vi "main_v1.1.vi"() -> ()   [LabVIEW 2012]
uses:
  SensorSettingCtl.ctl
  SensorTypes.ctl
  states.ctl
  globalVariables.vi
  <vilib>/Analysis/baseanly.llb/Mean (DBL).vi
  <vilib>/Analysis/NI_AALBase.lvlib
panel:
  in  "endindices":i32[](array[numeric])
  in  "startindices":i32[](array[numeric])
  in  "cancel button data analysis":bool
  out "XY Graph 11":cluster{dbl[], dbl[]}[](graph)
  out "XY Graph 10":cluster{dbl[], dbl[]}[](graph)
  out "size":i32[](array[numeric])
  out "sum":dbl[](array[numeric])
  out "XY Graph 9":cluster{dbl[], dbl[]}[](graph)
  out "XY Graph 8":cluster{dbl[], dbl[]}[](graph)
  out "meas. time / s":dbl format="%#.1f"
  out "diff chg":dbl
  out "charges":dbl[](array[numeric])
  out "times":dbl[](array[numeric])
  out "diff":dbl
  in  "max. meas. time / s":dbl=3000.0
  out "mean currents":dbl[](array[numeric])
  out "measuring":bool
  out "i_e":i32
  out "i_s":i32
  out "XY Graph raw":cluster{dbl[], dbl[]}[](graph)
  out "XY Graph":cluster{dbl[], dbl[]}[](graph)
  in  "size of buffer":i32=1000000
  in  "Path for measuring results":path=path "C:/Users/Induelec/Desktop/test_output"
  in  "Sensor types":T1[](array[typedef])=[enum."ITL 900 (Analogue)", enum."CAB 300-C SP3 (CAN)", enum."xyz TODO (PWM)", enum."xyz TODO (LIN)", enum."xyz TODO (Analogue)"]
  in  "Sensor-enabling":T2[](array[typedef])=[{"VISA resource name"="", "use sensor"=FALSE}, {"VISA resource name"="", "use sensor"=TRUE}, {"VISA resource name"="", "use sensor"=FALSE}, {"VISA resource name"="", "use sensor"=FALSE}, {"VISA resource name"="", "use sensor"=FALSE}]
  in  "cancel button":bool
  in  "start Button":bool
  out "Error Flag":bool
  # "Measurement of Current Sensors from LEM"
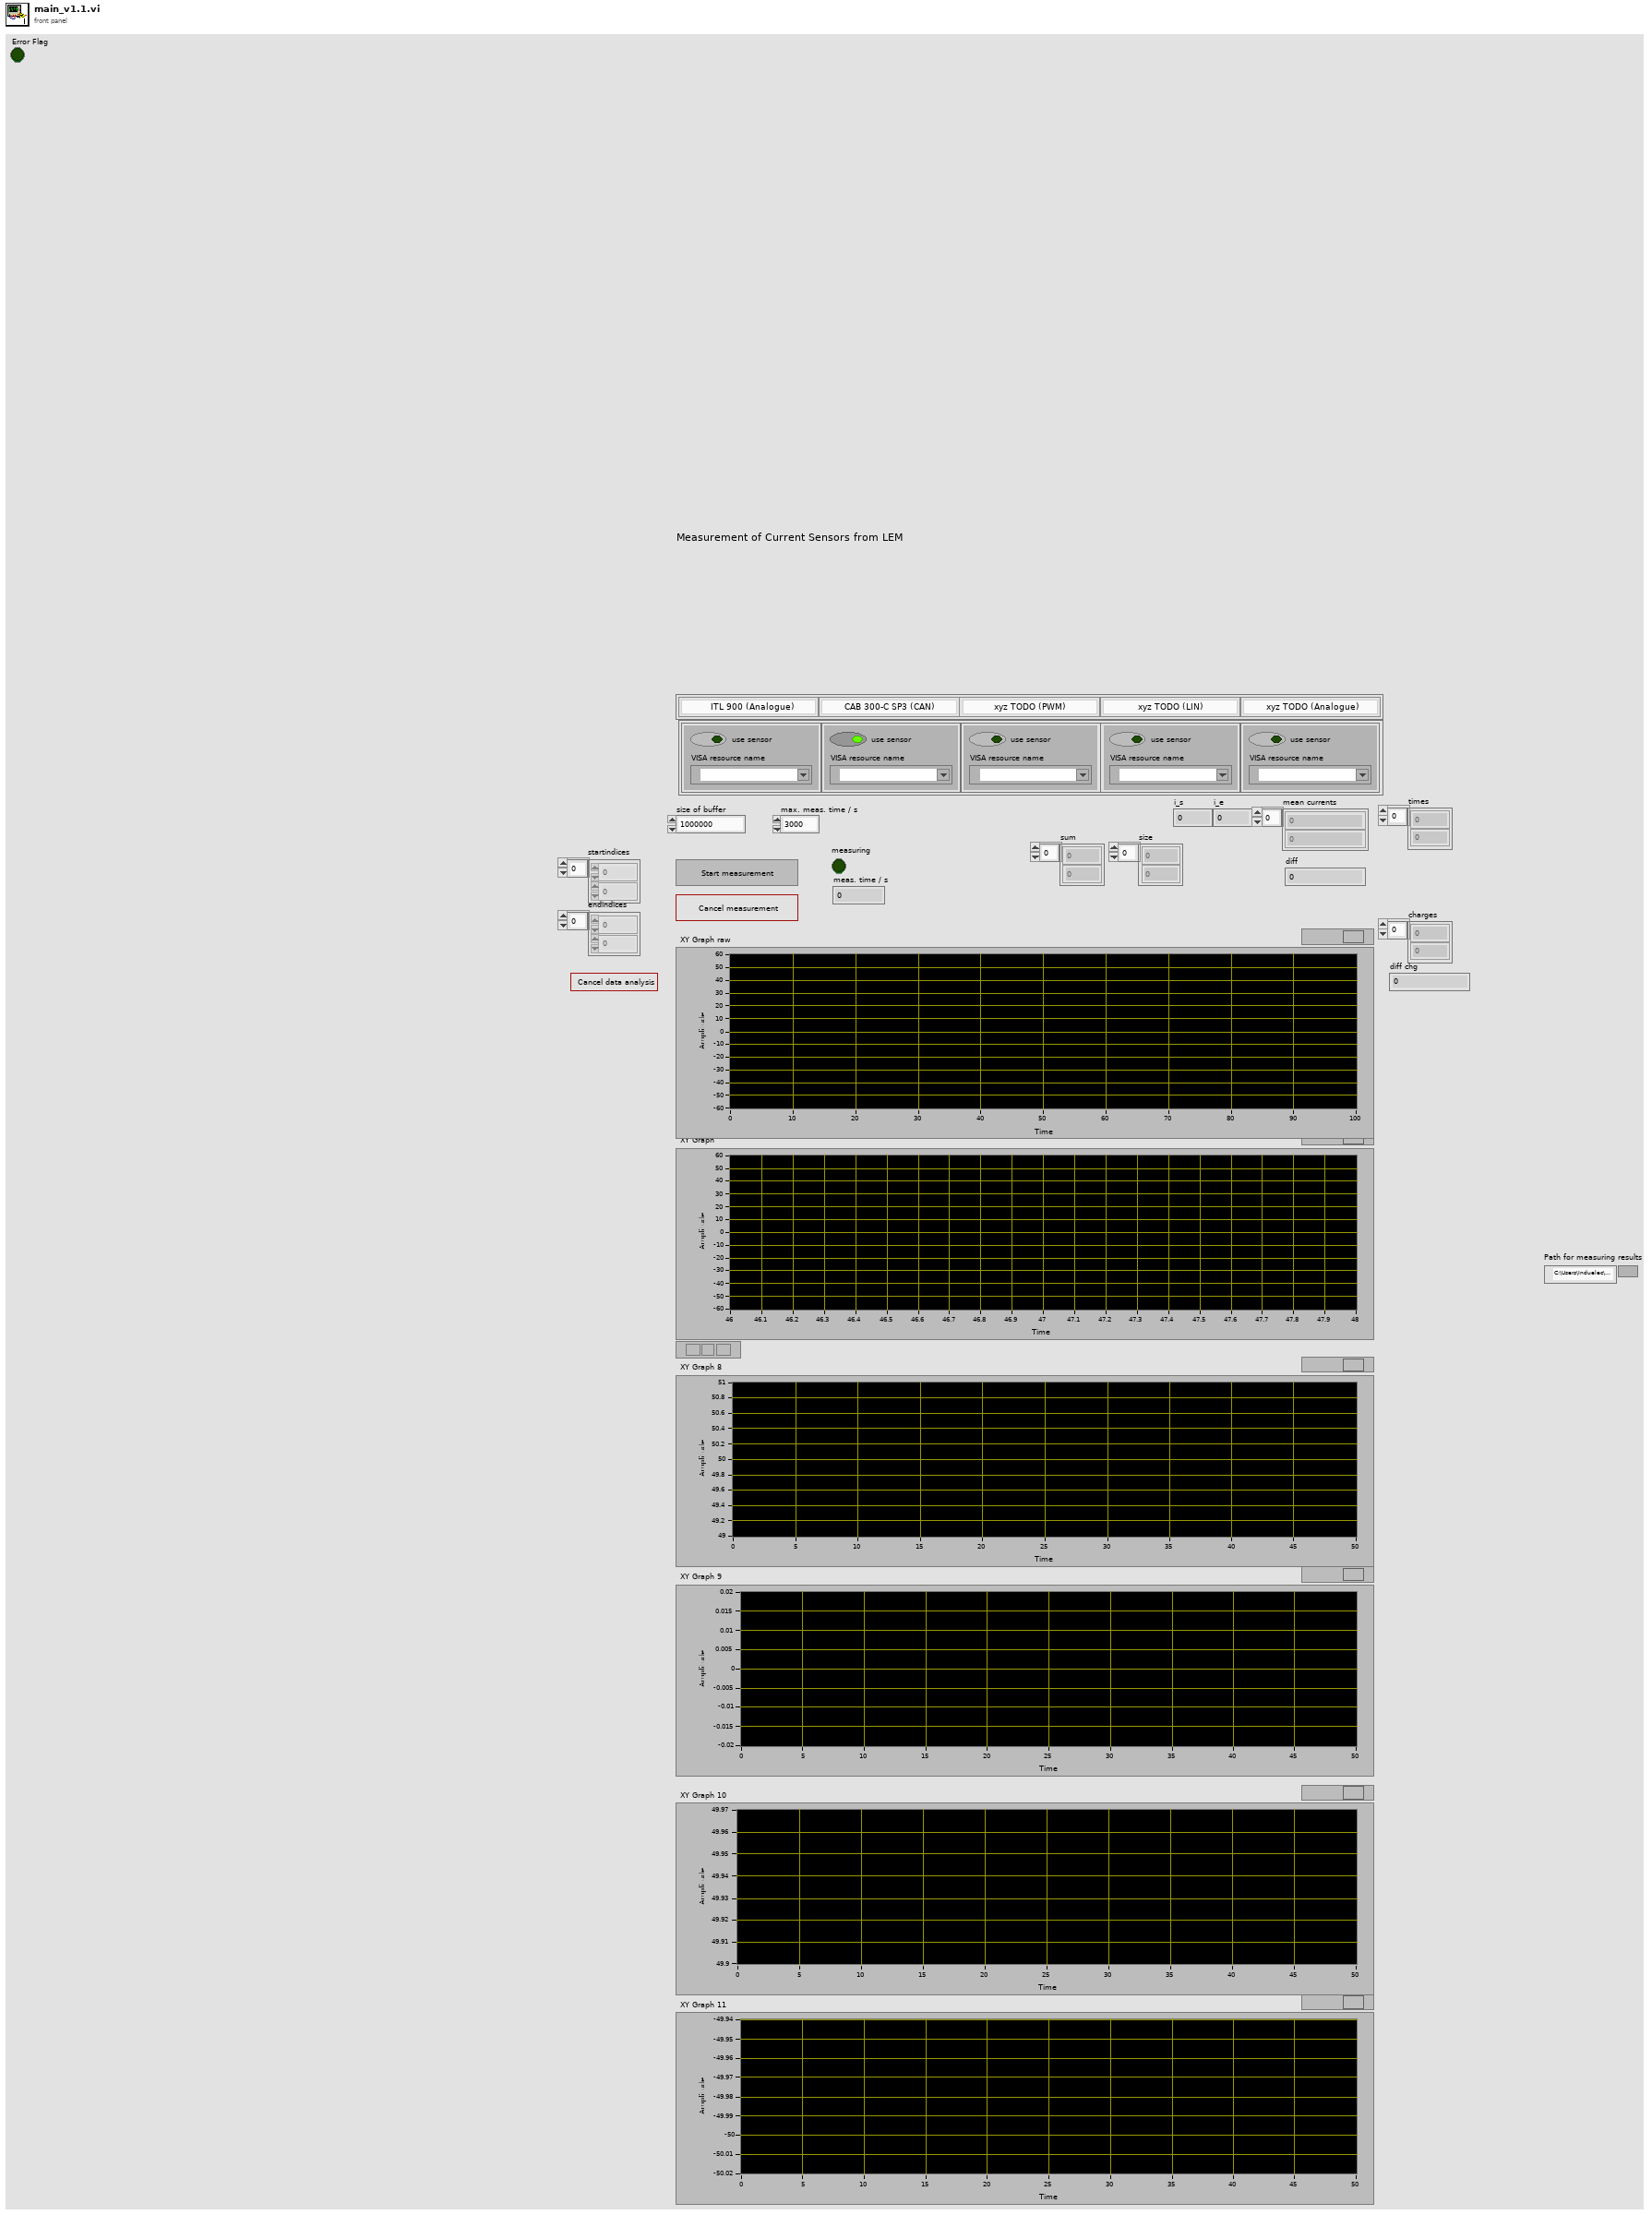
[diagram p1: front panel]
types:
  T1 = typedef "SensorTypes.ctl" = enum16{"ITL 900 (Analogue)", "CAB 300-C SP3 (CAN)", "xyz TODO (PWM)", "xyz TODO (LIN)", "xyz TODO (Analogue)"}
  T2 = typedef "SensorSettingCtl.ctl" = cluster{"VISA resource name":refnum<visa-resource-name>, "use sensor":bool}
  T3 = typedef "states.ctl" = enum16{"init", "wait for user confirm", "start sensors", "measure", "data analysis", "terminate"}
  T4 = typedef "Semaphore RefNum" = refnum<k1>
  T5 = typedef "TimeValue.ctl" = cluster{"Time of measurement":timestamp, "Current value":dbl}
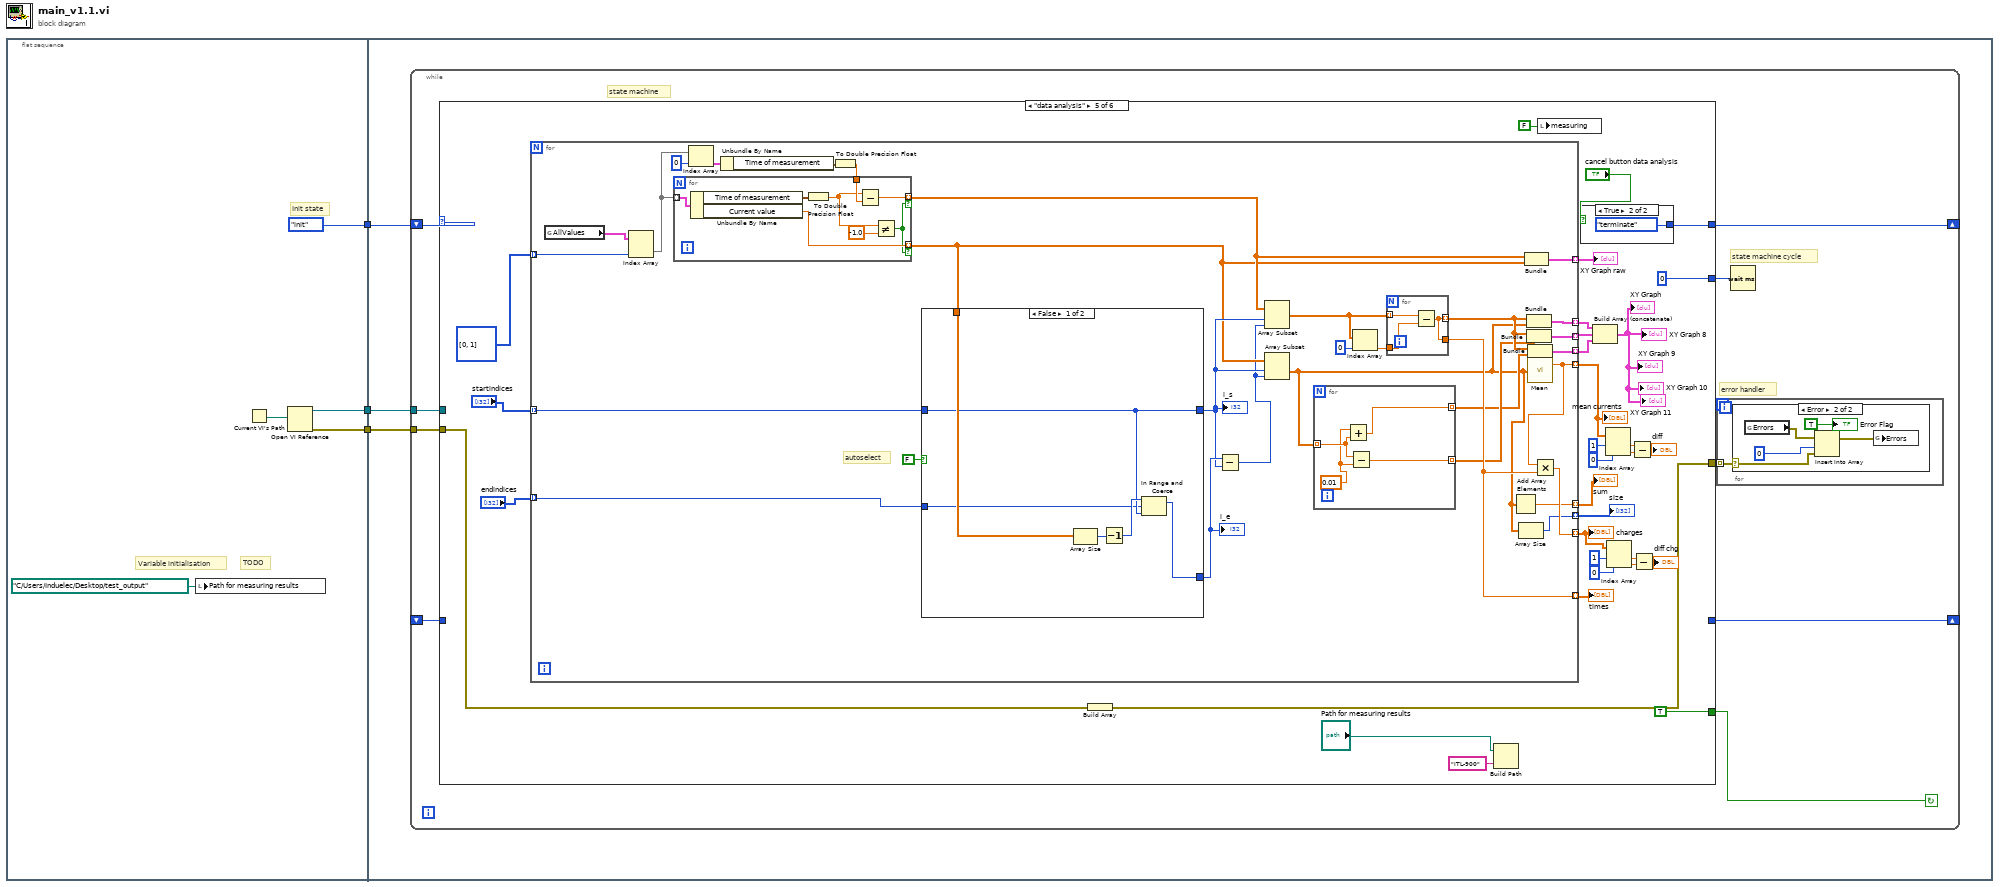
[diagram p0: block diagram]
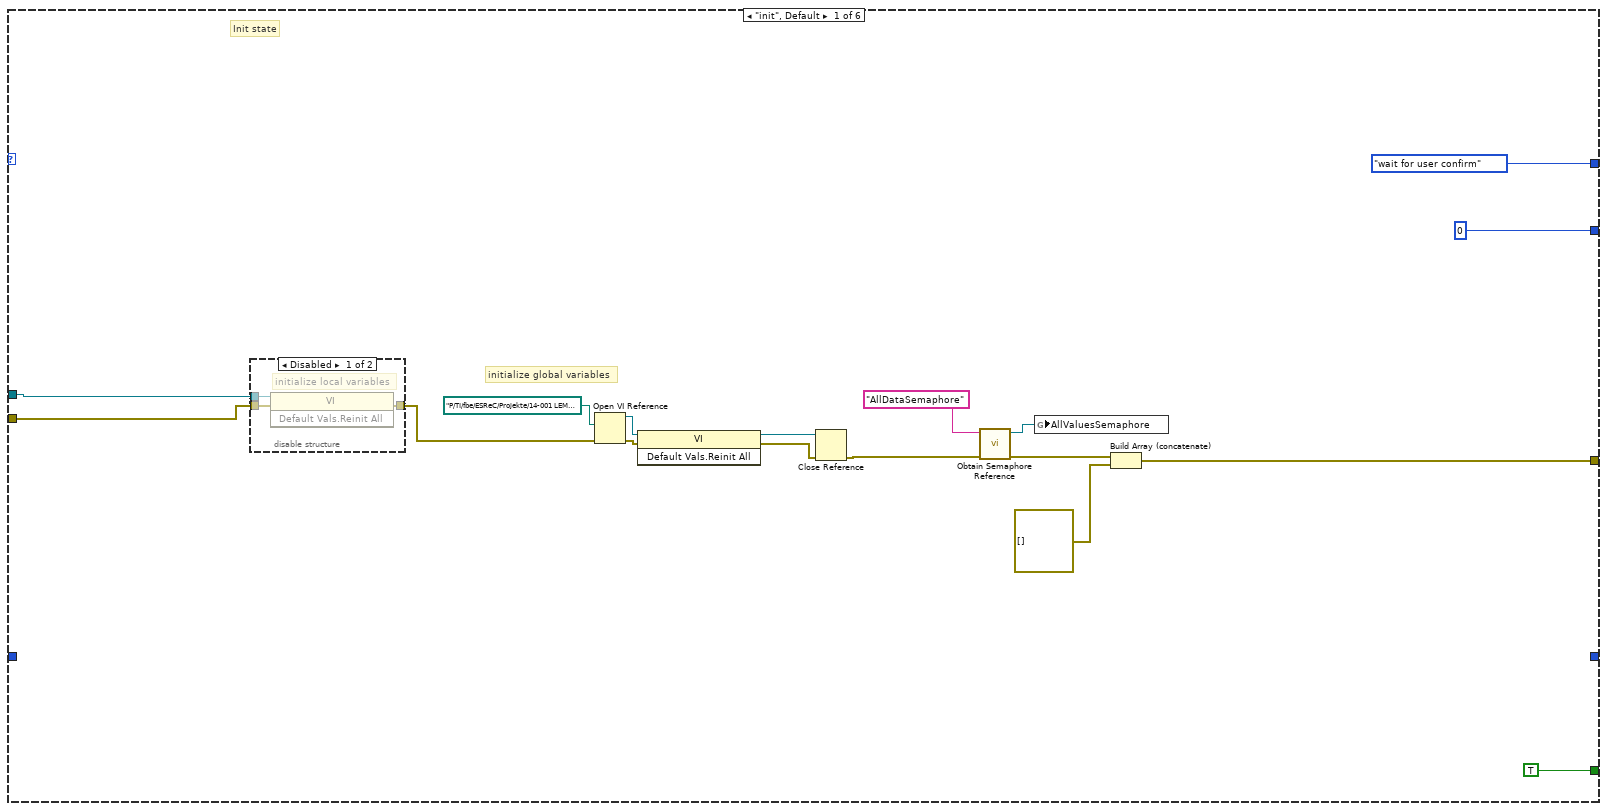
[diagram p3: hidden frame]
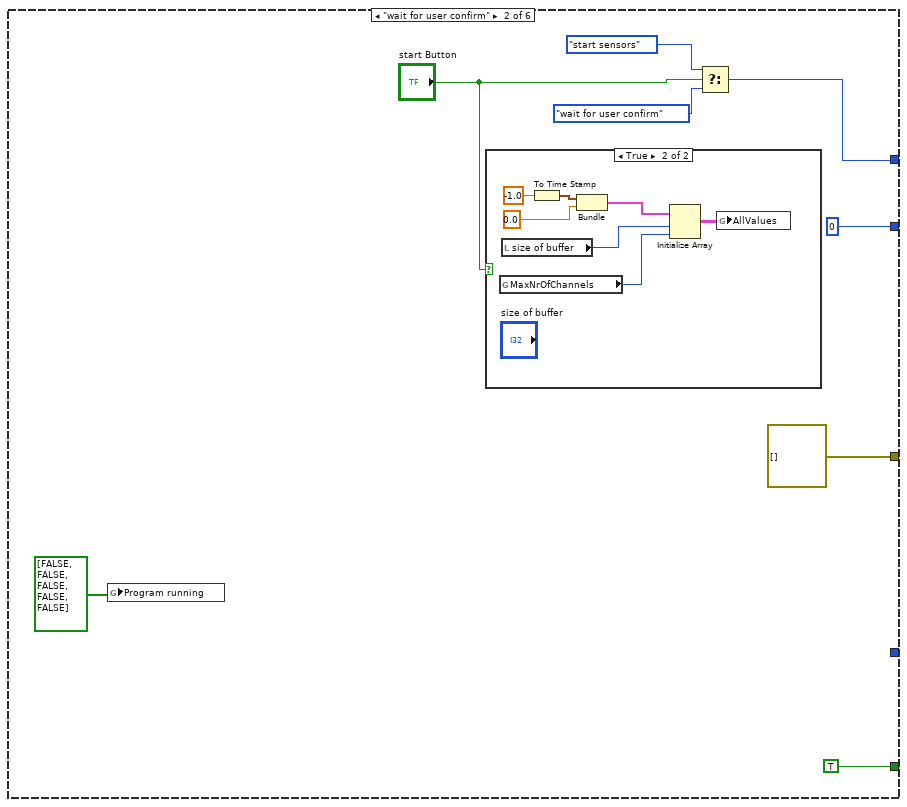
[diagram p5: hidden frame]
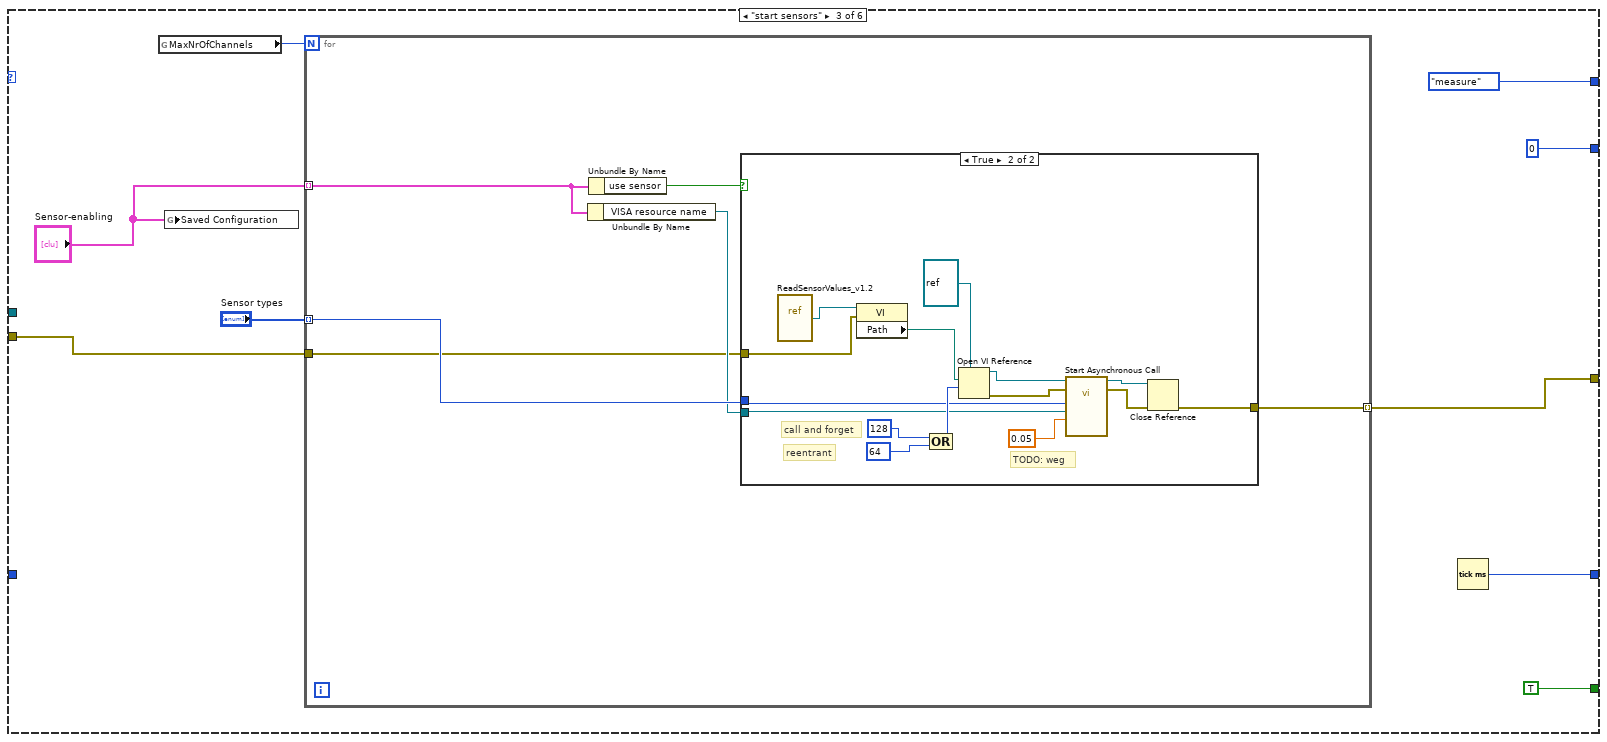
[diagram p7: hidden frame]
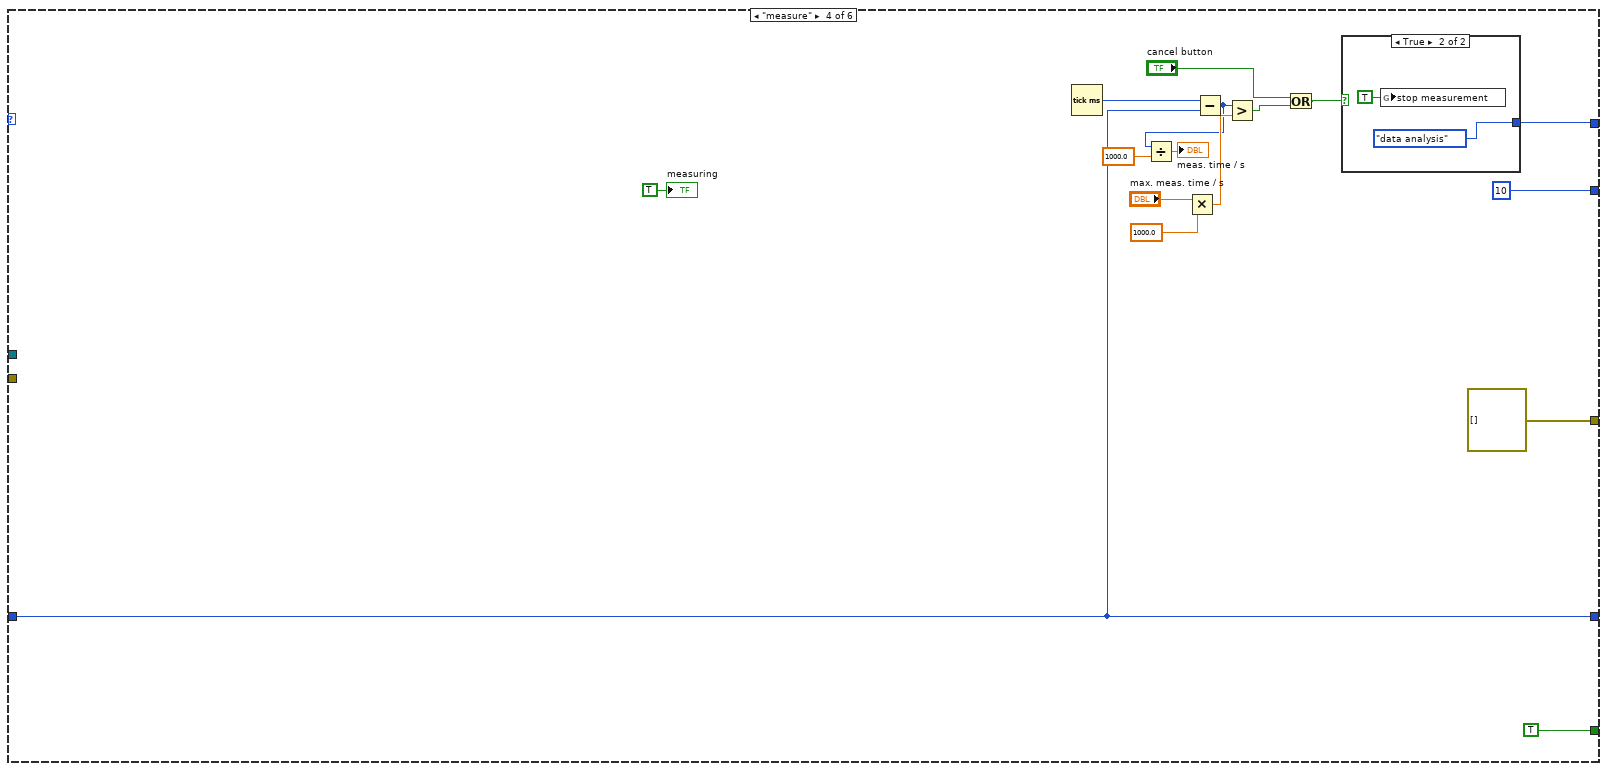
[diagram p9: hidden frame]
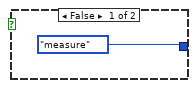
[diagram p10: hidden frame]
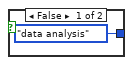
[diagram p11: hidden frame]
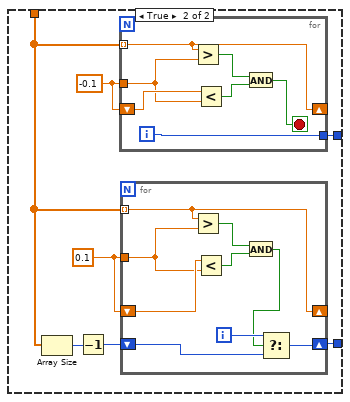
[diagram p12: hidden frame]
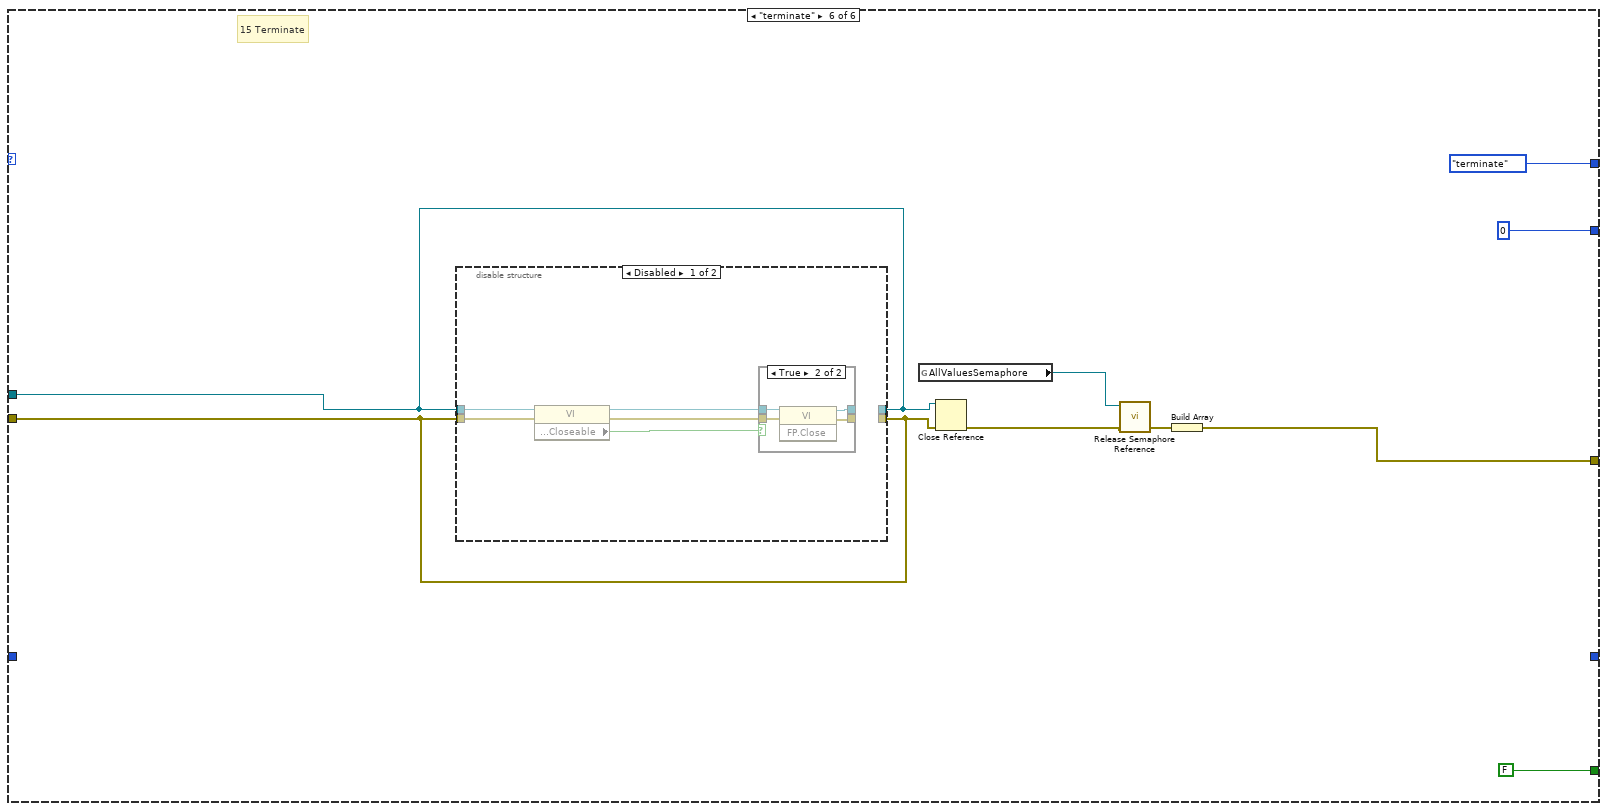
[diagram p13: hidden frame]
diagram:
  n1 = flat-sequence {
    tunnel: [states."init" ("States IEEE-488")] -> w3
    tunnel: [w8] -> w2
    tunnel: [w7] -> w1
    tunnel: w3 -> [w9]
    tunnel: w2 -> [w11]
    tunnel: w1 -> [w10]
    frame #0 {
      # "TODO"
      # "Variable initialisation"
      # "Init state"
      n2 = local write "Path for measuring results"(path "C:/Users/Induelec/Desktop/test_output" ("Path for measuring results")) -> ()
      n3 = Current VI's Path() -> (path=w6:path)
      n4 = Open VI Reference(vi path=w6) -> (vi reference=w8:refnum<vi>, error out=w7:errorcluster)  [unwired: 2 in, 3 out]
    }
    frame #1 {
      n5 = while {
        tunnel: w11 -> [w19]
        tunnel: w10 -> [w18]
        shift-right: [w15] -> _
        shift-left: w9 -> [w16]
        shift-right: [w13] -> _
        shift-left: _ -> [w12]
        stop <- w14 continue-if-true
        # "state machine"
        # "error handler"
        # "state machine cycle"
        n6 = case shown="\"data analysis\"" w16 {
          tunnel: [u32 0 ("milliseconds to wait") u32 0 ("milliseconds to wait") u32 0 ("milliseconds to wait") u32 10 ("milliseconds to wait") u32 0 ("milliseconds to wait") u32 0 ("milliseconds to wait")] -> w20
          tunnel: w19 -> [w40 _ _ _ _ w225]
          tunnel: w18 -> [w41 _ w63 _ w138 w224]
          tunnel: [w42 errorcluster[] [] w68 errorcluster[] [] w139 w228] -> w17
          tunnel: [states."wait for user confirm" ("States IEEE-488") w52 states."measure" ("States IEEE-488") w107 w140 states."terminate" ("f")] -> w15
          tunnel: [TRUE TRUE TRUE TRUE TRUE FALSE] -> w14
          tunnel: [_ _ w62 w101 _ _] -> w13
          tunnel: w12 -> [_ _ _ w101 _ _]
          frame "init", Default {
            # "initialize global variables"
            # "Init state"
            n7 = disable-structure shown="Disabled" {
              disable-tunnel: w41 -> [w46 _]
              disable-tunnel: w40 -> [w45 _]
              disable-tunnel: [w44 _] -> w34
              frame Disabled {
                # "initialize local variables"
                n8 = invoke class="VI" method="Default Vals.Reinit All"(reference=w45, error in=w46) -> (error out=w44:errorcluster)  [unwired: 1 in, 2 out]
              }
              frame Enabled {
              }
            }
            n9 = Open VI Reference(vi path=path "P:/TI/fbe/ESReC/Projekte/14-001 LEM Current Sensor Measurements/Software/LabVIEW/Current sensor tests/globalVariables.vi", error in (no error)=w34) -> (vi reference=w35:refnum<vi>, error out=w33:errorcluster)  [unwired: 4 in]
            n10 = invoke class="VI" method="Default Vals.Reinit All"(reference=w35, error in=w33) -> (reference out=w32:refnum<vi>, error out=w31:errorcluster)  [unwired: 1 in, 1 out]
            n11 = Close Reference(reference=w32, error in (no error)=w31) -> (error out=w29:errorcluster)
            n12 = call <vilib>:"Obtain Semaphore Reference.vi"("error in (no error)"=w29, "name (unnamed)"="AllDataSemaphore") -> ("error out"=w28:errorcluster, "semaphore"=w27:T4)  [unwired: 3 in, 1 out]
            n13 = global write "globalVariables.vi" "AllValuesSemaphore"(w27) -> ()
            n14 = Build Array (concatenate)(w28, errorcluster[] [] ("array")) -> (w42:errorcluster[])
          }
          frame "wait for user confirm" {
            n15 = global write "globalVariables.vi" "Program running"(bool[] [FALSE, FALSE, FALSE, FALSE, FALSE] ("Program running")) -> ()
            n16 = case shown="True" "start Button" {
              frame False {
              }
              frame True {
                n17 = global read "globalVariables.vi" "MaxNrOfChannels"() -> (w61:i32)
                n18 = local read "size of buffer"() -> (w59:i32)
                n19 = To Time Stamp(1:-1.0 ("number")) -> (0:w57:timestamp)
                n20 = Bundle(w57, 0.0) -> (w55:cluster{timestamp, dbl})  [unwired: 1 in]
                n21 = Initialize Array(w55, w59, w61) -> (w60:cluster{timestamp, dbl}[][])
                n22 = global write "globalVariables.vi" "AllValues"(w60) -> ()
              }
            }
            n23 = Select(t=states."start sensors" ("States IEEE-488"), s="start Button", f=states."wait for user confirm" ("States IEEE-488")) -> (s? t:f=w52:T3)
          }
          frame "start sensors" {
            n24 = global read "globalVariables.vi" "MaxNrOfChannels"() -> (w65:i32)
            n25 = global write "globalVariables.vi" "Saved Configuration"("Sensor-enabling") -> ()
            n26 = for {
              N: w65 -> [_]
              tunnel: "Sensor-enabling" -> [w75] mode=indexing
              tunnel: [w74] -> w68 mode=indexing
              tunnel: "Sensor types" -> [w73] mode=indexing
              tunnel: w63 -> [w71]
              n27 = Unbundle By Name(w75) -> ("VISA resource name"=w72:refnum<visa-resource-name>)
              n28 = Unbundle By Name(w75) -> ("use sensor"=w76:bool)
              n29 = case shown="True" w76 {
                tunnel: [w77 w90] -> w74
                tunnel: w73 -> [_ w83]
                tunnel: w72 -> [_ w82]
                tunnel: w71 -> [w77 w84]
                frame False {
                }
                frame True {
                  # "TODO: weg"
                  # "reentrant"
                  # "call and forget"
                  n30 = vi-ref "ReadSensorValues_v1.2.vi"() -> (w80:refnum<vi>)
                  n31 = property class="VI"(reference=w80, error in=w84) -> ("Path"=w92:path)  [unwired: 2 out]
                  n32 = Compound Arithmetic op=OR(128 ("options"), 64 ("value")) -> (w89:i32)
                  n33 = Open VI Reference(type specifier VI Refnum (for type only)=refnum<vi> refnum, vi path=w92, options=w89) -> (vi reference=w79:refnum<vi>, error out=w87:errorcluster)  [unwired: 3 in]
                  n34 = call-by-ref "Start Asynchronous Call"(reference=w79, error in=w87, "Sample time reference sensor / s"=0.05, "VISA resource name"=w82, "Sensor type"=w83) -> (reference out=w86:refnum<vi>, error out=w85:errorcluster)  [unwired: 1 in]
                  n35 = Close Reference(reference=w86, error in (no error)=w85) -> (error out=w90:errorcluster)
                }
              }
            }
            n36 = Tick Count (ms)() -> (millisecond timer value=w62:u32)
          }
          frame "measure" {
            n37 = Tick Count (ms)() -> (millisecond timer value=w95:u32)
            n38 = Multiply(x="max. meas. time / s", y=1000.0) -> (x*y=w98:dbl)
            n39 = Subtract(x=w95, y=w101) -> (x-y=w93:u32)
            n40 = Divide(x=w93, y=1000.0) -> (x/y=→"meas. time / s":dbl)
            n41 = Greater?(x=w93, y=w98) -> (0:w102:bool)
            n42 = Or(x="cancel button", y=w102) -> (x .or. y?=w104:bool)
            n43 = case shown="True" w104 {
              tunnel: [states."measure" ("f") states."data analysis" ("States IEEE-488")] -> w107
              frame False {
              }
              frame True {
                n44 = global write "globalVariables.vi" "stop measurement"(TRUE ("stop measurement")) -> ()
              }
            }
            "measuring" <- TRUE ("measuring")
          }
          frame "data analysis" {
            n45 = for {
              tunnel: [w171] -> w120 mode=indexing
              tunnel: i32[] [0, 1] -> [w170] mode=indexing
              tunnel: [w167] -> w135 mode=indexing
              tunnel: [w161] -> w133 mode=indexing
              tunnel: [w159] -> w129 mode=indexing
              tunnel: [w160] -> w121 mode=indexing
              tunnel: [w152] -> w119 mode=indexing
              tunnel: [w151] -> w118 mode=indexing
              tunnel: [w150] -> w117 mode=indexing
              tunnel: [w148] -> w116 mode=indexing
              tunnel: "startindices" -> [w147] mode=indexing
              tunnel: "endindices" -> [w146] mode=indexing
              # "autoselect"
              n46 = global read "globalVariables.vi" "AllValues"() -> (w176:T5[][])
              n47 = Index Array(array=w176, index (col)=w170) -> (element=w162:T5[])  [unwired: 1 in]
              n48 = Index Array(array=w162, index=0) -> (element=w174:T5)
              n49 = Unbundle By Name(w174) -> ("Time of measurement"=w173:timestamp)
              n50 = To Double Precision Float(number=w173) -> (double precision float=w172:dbl)
              n51 = for {
                tunnel: w162 -> [w220] mode=indexing
                tunnel: [w213] -> w166 mode=indexing if=w214
                tunnel: [w218] -> w158 mode=indexing if=w214
                tunnel: w172 -> [w217]
                n52 = Unbundle By Name(w220) -> ("Time of measurement"=w219:timestamp, "Current value"=w218:dbl)
                n53 = To Double Precision Float(number=w219) -> (double precision float=w215:dbl)
                n54 = Subtract(x=w215, y=w217) -> (x-y=w213:dbl)
                n55 = Not Equal?(x=w215, y=-1.0) -> (x != y?=w214:bool)
              }
              n56 = case shown="False" FALSE {
                tunnel: [w183 w191] -> w169
                tunnel: [w182 w190] -> w168
                tunnel: w158 -> [w185 w187]
                tunnel: w147 -> [w182 _]
                tunnel: w146 -> [w181 _]
                frame False {
                  n57 = Array Size(array=w185) -> (size(s)=w186:i32)
                  n58 = Decrement(x=w186) -> (x-1=w184:i32)
                  n59 = In Range and Coerce(upper limit=w184, x=w181, lower limit=w182) -> (coerced(x)=w183:i32)  [unwired: 1 out]
                }
                frame True {
                  w188 = -0.1
                  w189 = 0.1
                  n60 = Array Size(array=w187) -> (size(s)=w193:i32)
                  n61 = Decrement(x=w193) -> (x-1=w192:i32)
                  n62 = for {
                    tunnel: w187 -> [w205] mode=indexing
                    tunnel: [w209] -> w190
                    shift-right: [w205] -> _
                    shift-left: w188 -> [w204]
                    tunnel: w188 -> [w203]
                    i -> [w209]
                    stop <- w207 stop-if-true
                    n63 = Greater?(x=w205, y=w203) -> (0:w206:bool)
                    n64 = Less?(x=w204, y=w203) -> (x < y?=w208:bool)
                    n65 = And(x=w206, y=w208) -> (x .and. y?=w207:bool)
                  }
                  n66 = for {
                    tunnel: w187 -> [w196] mode=indexing
                    shift-right: [w202] -> w191
                    shift-left: w192 -> [w200]
                    shift-right: [w196] -> _
                    shift-left: w189 -> [w195]
                    tunnel: w189 -> [w194]
                    i -> [w201]
                    n67 = Greater?(x=w196, y=w194) -> (0:w199:bool)
                    n68 = Less?(x=w195, y=w194) -> (x < y?=w198:bool)
                    n69 = And(x=w199, y=w198) -> (x .and. y?=w197:bool)
                    n70 = Select(t=w201, s=w197, f=w200) -> (s? t:f=w202:i32)
                  }
                }
              }
              "i_s" <- w168
              "i_e" <- w169
              n71 = Subtract(x=w169, y=w168) -> (x-y=w156:i32)
              n72 = Array Subset(array=w166, index=w168, length=w156) -> (w165:dbl[])
              n73 = Array Subset(array=w158, index=w168, length=w156) -> (w149:dbl[])
              n74 = for {
                tunnel: w149 -> [w180] mode=indexing
                tunnel: [w178] -> w154 mode=indexing
                tunnel: [w177] -> w153 mode=indexing
                w179 = 0.01
                n75 = Add(x=w179, y=w180) -> (x+y=w177:dbl)
                n76 = Subtract(x=w180, y=w179) -> (x-y=w178:dbl)
              }
              n77 = Index Array(array=w165, index=0) -> (element=w163:dbl)
              n78 = for {
                tunnel: w165 -> [w212] mode=indexing
                tunnel: w163 -> [w211]
                tunnel: [w210] -> w155 mode=indexing
                tunnel: [w210] -> w159
                n79 = Subtract(x=w212, y=w211) -> (x-y=w210:dbl)
              }
              n80 = Add Array Elements(numeric array=w149) -> (sum=w150:dbl)
              n81 = Array Size(array=w149) -> (size(s)=w148:i32)
              n82 = Bundle(w166, w158) -> (w167:cluster{dbl[], dbl[]})  [unwired: 1 in]
              n83 = Bundle(w155, w149) -> (w171:cluster{dbl[], dbl[]})  [unwired: 1 in]
              n84 = Bundle(w155, w154) -> (w152:cluster{dbl[], dbl[]})  [unwired: 1 in]
              n85 = Bundle(w155, w153) -> (w151:cluster{dbl[], dbl[]})  [unwired: 1 in]
              n86 = call-poly <vilib>:"Mean.vi"("X"=w149) -> ("mean"=w161:dbl)  [unwired: 1 out]
              n87 = Multiply(x=w161, y=w159) -> (x*y=w160:dbl)
            }
            "XY Graph raw" <- w135
            "mean currents" <- w133
            "times" <- w129
            "charges" <- w121
            "sum" <- w117
            "size" <- w116
            n88 = Build Array(w138) -> (w139:errorcluster[])
            n89 = Build Path(base path="Path for measuring results", name or relative path="ITL-900") -> ()  [unwired: 1 out]
            n90 = local write "measuring"(FALSE ("measuring")) -> ()
            n91 = case shown="True" "cancel button data analysis" {
              tunnel: [states."data analysis" ("f") states."terminate" ("f")] -> w140
              frame False {
              }
              frame True {
              }
            }
            n92 = Build Array (concatenate)(w120, w119, w118) -> (→"XY Graph" →"XY Graph 8" →"XY Graph 9" →"XY Graph 10" →"XY Graph 11":cluster{dbl[], dbl[]}[])
            n93 = Index Array(array=w133, index #1=1 ("index"), index #2=0 ("index")) -> (element #1=w131:dbl, element #2=w130:dbl)
            n94 = Index Array(array=w121, index #1=1 ("index"), index #2=0 ("index")) -> (element #1=w123:dbl, element #2=w124:dbl)
            n95 = Subtract(x=w131, y=w130) -> (x-y=→"diff":dbl)
            n96 = Subtract(x=w123, y=w124) -> (x-y=→"diff chg":dbl)
          }
          frame "terminate" {
            # "15 Terminate"
            n97 = disable-structure shown="Disabled" {
              disable-tunnel: w224 -> [w231 _]
              disable-tunnel: w225 -> [w230 _]
              disable-tunnel: w225 -> [_ _]
              disable-tunnel: w224 -> [_ _]
              frame Disabled {
                n98 = property class="VI"(reference=w230, error in=w231) -> (reference out=w233:refnum<vi>, error out=w232:errorcluster, "Front Panel.Closeable"=w234:bool)
                n99 = case shown="True" w234 {
                  tunnel: w233 -> [w236 w240]
                  tunnel: [w236 w239] -> _
                  tunnel: w232 -> [w235 w238]
                  tunnel: [w235 w237] -> _
                  frame False {
                  }
                  frame True {
                    n100 = invoke class="VI" method="FP.Close"(reference=w240, error in=w238) -> (reference out=w239:refnum<vi>, error out=w237:errorcluster)  [unwired: 1 in, 1 out]
                  }
                }
              }
              frame Enabled {
              }
            }
            n101 = global read "globalVariables.vi" "AllValuesSemaphore"() -> (w221:T4)
            n102 = Close Reference(reference=w225, error in (no error)=w224) -> (error out=w223:errorcluster)
            n103 = call <vilib>:"Release Semaphore Reference.vi"("error in (no error)"=w223, "semaphore"=w221) -> ("error out"=w222:errorcluster)  [unwired: 8 in, 1 out]
            n104 = Build Array(w222) -> (w228:errorcluster[])
          }
        }
        n105 = for {
          tunnel: w17 -> [w21] mode=indexing
          n106 = case shown="Error" w21 {
            selector: w21 -> [_ w25]
            frame No Error {
            }
            frame Error {
              n107 = global read "globalVariables.vi" "Errors"() -> (w23:errorcluster[])
              n108 = Insert Into Array(array=w23, index=0, new element=w25) -> (w22:errorcluster[])
              n109 = global write "globalVariables.vi" "Errors"(w22) -> ()
              "Error Flag" <- TRUE ("Error Flag")
            }
          }
        }
        n110 = Wait (ms)(milliseconds to wait=w20) -> ()  [unwired: 1 out]
      }
    }
  }
